vi "HRmax calculate.vi"(8 "error in":errorcluster, 10 "Age":u8, 11 "Sex":enum16{"Male", "Female"}(ring)) -> (0 "error out":errorcluster, 3 "HR Max":dbl)   [LabVIEW 2016]
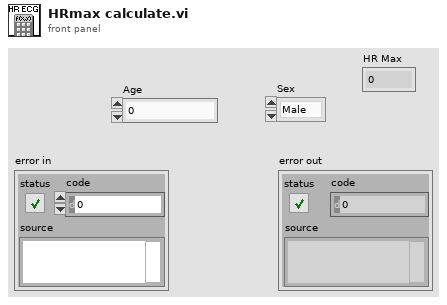
[diagram p1: front panel]
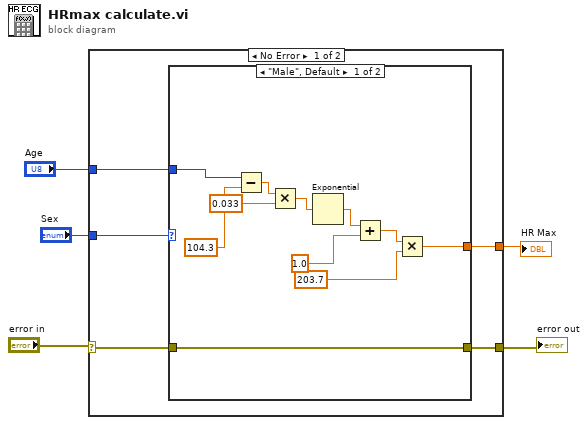
[diagram p0: block diagram]
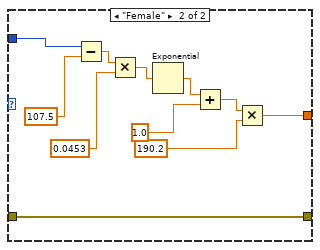
[diagram p2: hidden frame]
diagram:
  n1 = case shown="No Error" "error in" {
    selector: "error in" -> [w9 w33]
    tunnel: "Sex" -> [w10 _]
    tunnel: "Age" -> [w8 _]
    tunnel: [w7 _] -> w2
    tunnel: [w6 w33] -> w1
    frame No Error {
      n2 = case shown="\"Male\", Default" w10 {
        tunnel: w9 -> [w11 w22]
        tunnel: w8 -> [w21 w24]
        tunnel: [w12 w23] -> w7
        tunnel: [w11 w22] -> w6
        frame "Male", Default {
          n3 = Subtract(x=w21, y=104.3) -> (x-y=w19:dbl)
          n4 = Multiply(x=w19, y=0.033) -> (x*y=w17:dbl)
          n5 = Exponential(1:w17) -> (0:w16:dbl)
          n6 = Add(x=w16, y=1.0) -> (x+y=w14:dbl)
          n7 = Multiply(x=w14, y=203.7) -> (x*y=w12:dbl)
        }
        frame "Female" {
          n8 = Subtract(x=w24, y=107.5) -> (x-y=w31:dbl)
          n9 = Multiply(x=w31, y=0.0453) -> (x*y=w29:dbl)
          n10 = Exponential(1:w29) -> (0:w28:dbl)
          n11 = Add(x=w28, y=1.0) -> (x+y=w26:dbl)
          n12 = Multiply(x=w26, y=190.2) -> (x*y=w23:dbl)
        }
      }
    }
    frame Error {
    }
  }
  "error out" <- w1
  "HR Max" <- w2
